vi "Initialize Device.vi"(7 "Baud Rate Override":u32, 8 "Error In":errorcluster, 9 "TCP Configuration":T3, 10 "COM Port":refnum<visa-resource-name>, 11 "Interface":T2) -> (0 "Error Out":errorcluster, 2 "Device Name":string, 3 "LINX Device Config":T1)   [LabVIEW 2011, in "LVH-LINX.lvlib" / "Device.lvlib"]
doc: "Open a connection to the LINX device."
uses:
  Device.lvlib
  Type Defs/TCP Config.ctl
  Type Defs/Interface.ctl
  Type Defs/LINX Device Config.ctl
  Type Defs/Device Family.ctl
  Type Defs/Channels.ctl
  Type Defs/Packet Number FGV Action.ctl
  LVH-LINX.lvlib
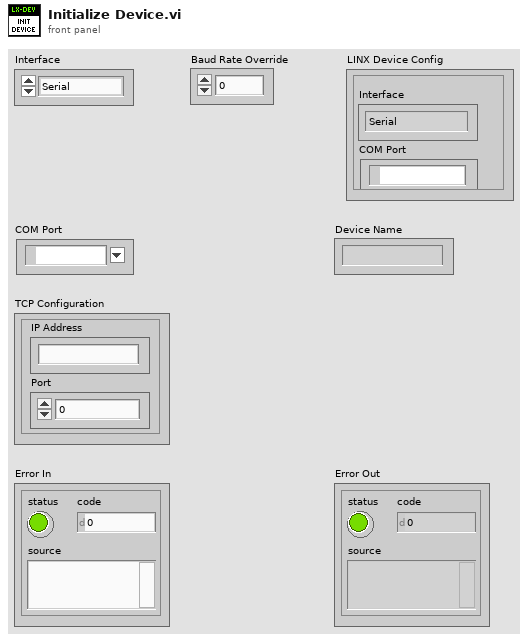
[diagram p1: front panel]
types:
  T1 = typedef "LVH-LINX.lvlib/Device.lvlib/LINX Device Config.ctl" = cluster{"Interface":T2, "COM Port":refnum<visa-resource-name>, "TCP Configuration":T3, "Device Family":T4, "Device ID":u8, "Device Name":string, "TCP Ref":refnum<k5>, "Channels":T5}
  T2 = typedef "LVH-LINX.lvlib/Interface.ctl" = enum16{"Serial", "TCP"}
  T3 = typedef "LVH-LINX.lvlib/Device.lvlib/TCP Config.ctl" = cluster{"IP Address":string, "Port":u16}
  T4 = typedef "LVH-LINX.lvlib/Device Family.ctl" = enum8{"National Instruments", "Digilent", "Arduino"}
  T5 = typedef "LVH-LINX.lvlib/Channels.ctl" = cluster{"DI Channels":u8[], "DO Channels":u8[], "AI":u8[], "AO":u8[], "PWM":u8[], "QE":u8[], "UART":u8[], "I2C 2":u8[], "SPI":u8[], "CAN":u8[], "AI Ref (V)":dbl, "AO Resolution (Bits)":u8, "AO Ref (V)":dbl}
  T6 = typedef "LVH-LINX.lvlib/Device.lvlib/Packet Number FGV Action.ctl" = enum16{"Initialize", "Get", "Increment"}
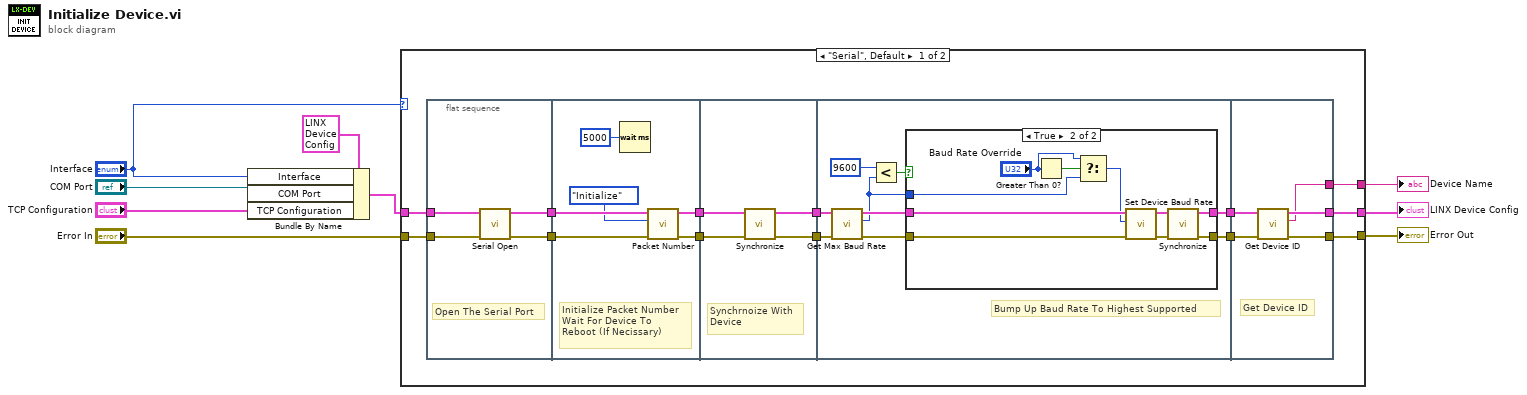
[diagram p0: block diagram]
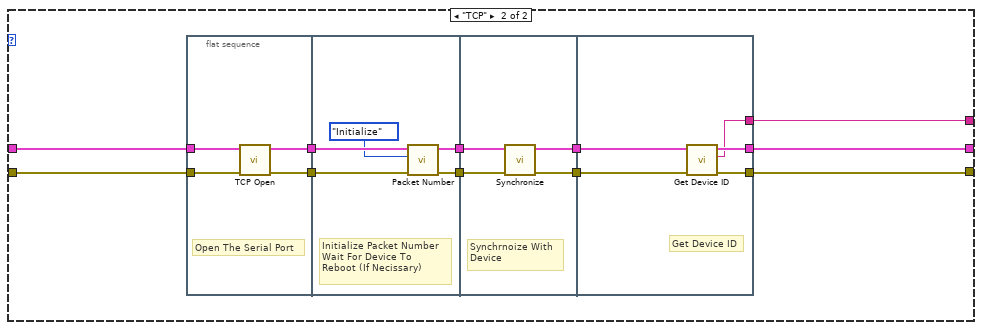
[diagram p3: hidden frame]
diagram:
  n1 = Bundle By Name(cluster=T1 {"Interface"=enum."Serial", "COM Port"="", "TCP Configuration"={"IP Address"="", "Port"=0}, "Device Family"=enum."National Instruments", "Device ID"=0, "Device Name"="", "TCP Ref"=refnum, "Channels"={"DI Channels"=[], "DO Channels"=[], "AI"=[], "AO"=[], "PWM"=[], "QE"=[], "UART"=[], "I2C 2"=[], "SPI"=[], "CAN"=[], "AI Ref (V)"=0.0, "AO Resolution (Bits)"=0, "AO Ref (V)"=0.0}} ("LINX Device Config"), "Interface"="Interface", "COM Port"="COM Port", "TCP Configuration"="TCP Configuration") -> (w4:T1)
  n2 = case shown="\"Serial\", Default" "Interface" {
    tunnel: "Error In" -> [w22 w73]
    tunnel: [w15 w66] -> w2
    tunnel: w4 -> [w21 w72]
    tunnel: [w16 w67] -> w3
    tunnel: [w10 w63] -> w1
    frame "Serial", Default {
      n3 = flat-sequence {
        tunnel: w22 -> [w26]
        tunnel: w21 -> [w25]
        tunnel: [w24] -> w20
        tunnel: [w23] -> w17
        tunnel: w20 -> [w30]
        tunnel: [w29] -> w19
        tunnel: [w28] -> w18
        tunnel: w17 -> [w31]
        tunnel: w19 -> [w36]
        tunnel: w18 -> [w35]
        tunnel: [w34] -> w14
        tunnel: [w33] -> w13
        tunnel: w14 -> [w45]
        tunnel: w13 -> [w44]
        tunnel: [w39] -> w12
        tunnel: [w38] -> w11
        tunnel: [w60] -> w15
        tunnel: [w61] -> w16
        tunnel: w12 -> [w62]
        tunnel: w11 -> [w59]
        tunnel: [w58] -> w10
        frame #0 {
          # "Open The Serial Port"
          n4 = call "Serial Open.vi"("Error In"=w26, "LINX Device Config"=w25) -> ("Error Out"=w23:errorcluster, "LINX Device Config"=w24:T1)  [unwired: 8 in]
        }
        frame #1 {
          # "Initialize Packet Number\nWait For Device To \nReboot (If Necissary)"
          n5 = Wait (ms)(milliseconds to wait=u32 5000) -> ()  [unwired: 1 out]
          n6 = call "Packet Number.vi"("Error In"=w31, "Action"=Packet_Number_FGV_Action."Initialize", "LINX Device Config"=w30) -> ("Error Out"=w28:errorcluster, "LINX Device Config"=w29:T1)  [unwired: 6 in, 1 out]
        }
        frame #2 {
          # "Synchrnoize With\nDevice"
          n7 = call "Synchronize.vi"("Error In"=w35, "LINX Device Config"=w36) -> ("Error Out"=w33:errorcluster, "LINX Device Config"=w34:T1)  [unwired: 8 in]
        }
        frame #3 {
          # "Bump Up Baud Rate To Highest Supported"
          n8 = call "Get Max Baud Rate.vi"("Error In"=w44, "LINX Device Config"=w45) -> ("Error Out"=w42:errorcluster, "Baud Rate"=w37:u32, "LINX Device Config"=w43:T1)  [unwired: 7 in]
          n9 = Less?(x=u32 9600 ("y"), y=w37) -> (x < y?=w40:bool)
          n10 = case shown="True" w40 {
            tunnel: w43 -> [w47 w57]
            tunnel: w42 -> [w46 w56]
            tunnel: [w47 w53] -> w39
            tunnel: [w46 w52] -> w38
            tunnel: w37 -> [_ w49]
            frame False {
              # "No Faster Baud Rates Supported"
            }
            frame True {
              n11 = Greater Than 0?(x="Baud Rate Override") -> (x > 0?=w50:bool)
              n12 = Select(t="Baud Rate Override", s=w50, f=w49) -> (s? t:f=w48:u32)
              n13 = call "Set Device Baud Rate.vi"("Error In"=w56, "Baud Rate"=w48, "LINX Device Config"=w57) -> ("Error Out"=w54:errorcluster, "LINX Device Config"=w55:T1)  [unwired: 6 in, 1 out]
              n14 = call "Synchronize.vi"("Error In"=w54, "LINX Device Config"=w55) -> ("Error Out"=w52:errorcluster, "LINX Device Config"=w53:T1)  [unwired: 8 in]
            }
          }
        }
        frame #4 {
          # "Get Device ID"
          n15 = call "Get Device ID.vi"("Error In"=w59, "LINX Device Config"=w62) -> ("Error Out"=w60:errorcluster, "Device Name"=w58:string, "LINX Device Config"=w61:T1)  [unwired: 7 in]
        }
      }
    }
    frame "TCP" {
      n16 = flat-sequence {
        tunnel: w73 -> [w77]
        tunnel: w72 -> [w76]
        tunnel: [w75] -> w71
        tunnel: [w74] -> w68
        tunnel: w71 -> [w81]
        tunnel: [w80] -> w70
        tunnel: [w79] -> w69
        tunnel: w68 -> [w82]
        tunnel: w70 -> [w86]
        tunnel: w69 -> [w85]
        tunnel: [w84] -> w65
        tunnel: [w83] -> w64
        tunnel: [w90] -> w66
        tunnel: [w91] -> w67
        tunnel: w65 -> [w89]
        tunnel: w64 -> [w88]
        tunnel: [w87] -> w63
        frame #0 {
          # "Open The Serial Port"
          n17 = call "TCP Open.vi"("Error In"=w77, "LINX Device Config"=w76) -> ("Error Out"=w74:errorcluster, "LINX Device Config"=w75:T1)  [unwired: 8 in]
        }
        frame #1 {
          # "Initialize Packet Number\nWait For Device To \nReboot (If Necissary)"
          n18 = call "Packet Number.vi"("Error In"=w82, "Action"=Packet_Number_FGV_Action."Initialize", "LINX Device Config"=w81) -> ("Error Out"=w79:errorcluster, "LINX Device Config"=w80:T1)  [unwired: 6 in, 1 out]
        }
        frame #2 {
          # "Synchrnoize With\nDevice"
          n19 = call "Synchronize.vi"("Error In"=w85, "LINX Device Config"=w86) -> ("Error Out"=w83:errorcluster, "LINX Device Config"=w84:T1)  [unwired: 8 in]
        }
        frame #3 {
          # "Get Device ID"
          n20 = call "Get Device ID.vi"("Error In"=w88, "LINX Device Config"=w89) -> ("Error Out"=w90:errorcluster, "Device Name"=w87:string, "LINX Device Config"=w91:T1)  [unwired: 7 in]
        }
      }
    }
  }
  "Error Out" <- w2
  "LINX Device Config" <- w3
  "Device Name" <- w1
